vi "Update Cluster.vi"(7 "Element to Update":enum16{"<None>", "Name", "Age", "Is Married?"}(ring)=enum."Age", 8 "Is Married?":bool, 9 "Age":u8=23, 10 "Name":string="Adam", 11 "Customer Data in":cluster{}) -> (3 "Customer Data out":cluster{})   [LabVIEW 2019]
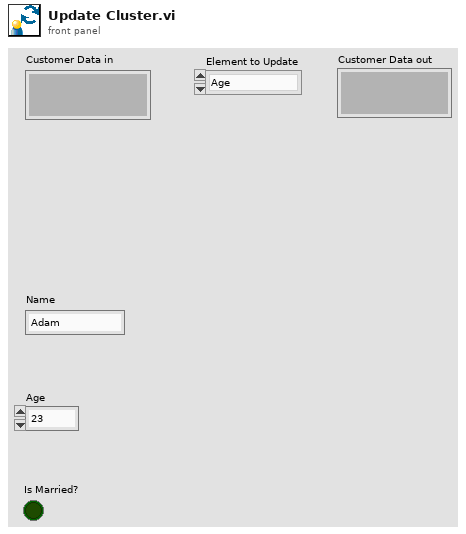
[diagram p1: front panel]
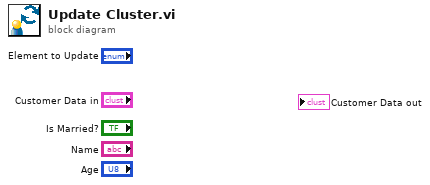
[diagram p0: block diagram]
diagram:
